vi "Update VI List.vi"(8 "error in (no error)":errorcluster, 10 "VI Infomation":T1[](array[typedef]), 11 "ViewController in":refnum<class "ViewController.lvclass">) -> (0 "error out":errorcluster, 3 "ViewController out":refnum<class "ViewController.lvclass">)   [LabVIEW 2018, in "ViewController.lvlib" / "ViewController.lvclass"]
uses:
  ViewController.lvclass
  Interface/Controls/VI Infomation.ctl
  ViewController.lvclass/ViewController.ctl
  Interface/Interface.lvlib
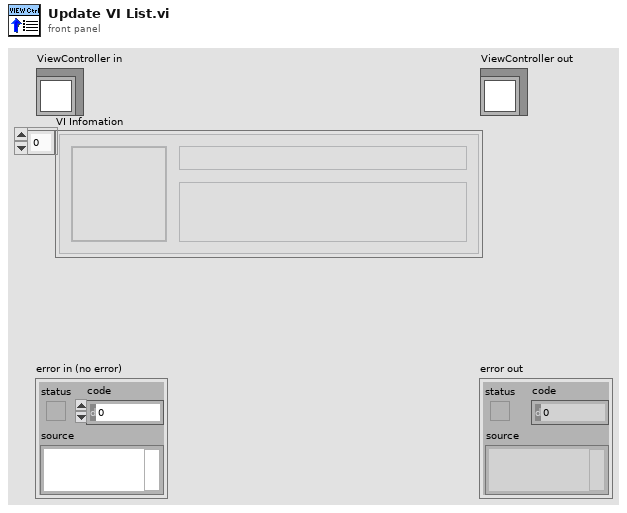
[diagram p1: front panel]
types:
  T1 = typedef "Interface.lvlib/VI Infomation.ctl" = cluster{"VI Name":string, "VI Description":string, "VI Icon":picture}
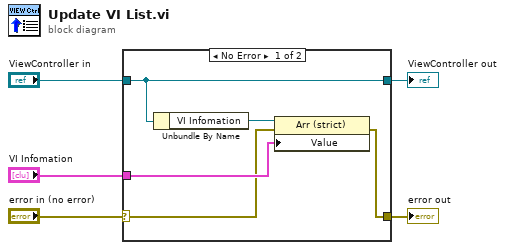
[diagram p0: block diagram]
diagram:
  n1 = case shown="No Error" "error in (no error)" {
    selector: "error in (no error)" -> [w7 w12]
    tunnel: "ViewController in" -> [w10 w11]
    tunnel: "VI Infomation" -> [w8 _]
    tunnel: [w6 w12] -> w2
    tunnel: [w10 w11] -> w1
    frame No Error {
      n2 = Unbundle By Name(w10) -> ("VI Infomation"=w9:refnum<vi>)
      n3 = property class="Arr (strict)"(reference=w9, error in=w7, "Value"=w8) -> (error out=w6:errorcluster)  [unwired: 1 out]
    }
    frame Error {
    }
  }
  "error out" <- w2
  "ViewController out" <- w1
